vi "Test Repetitive Calls to Next Differnet if Skip.vi"(8 "error in (no error)":errorcluster, 11 "Test Case In":refnum<class "Runnable Next Test.lvclass">) -> (0 "error out":errorcluster, 3 "Test Case Out":refnum<class "Runnable Next Test.lvclass">)   [LabVIEW 2020, in "Runnable Next Test.lvclass"]
uses:
  Runnable Next Test.lvclass
  Runnable Next Test.lvclass/Runnable Next Test.ctl
  Test Doubles/Test Case Test Double/Test Case Test Double.lvclass
  Test Doubles/Test Case Test Double/Methods.ctl
  source/API/LUnit Test Suite/LUnit Test Suite.lvclass
  59278e4f-a81c-4e4b-9980-f8e3984e3fef.vi
  source/API/LUnit Test Case/LUnit Test Case.lvclass
  C:/git/astemes-lunit/source/Core/Runnable/Runnable.lvclass
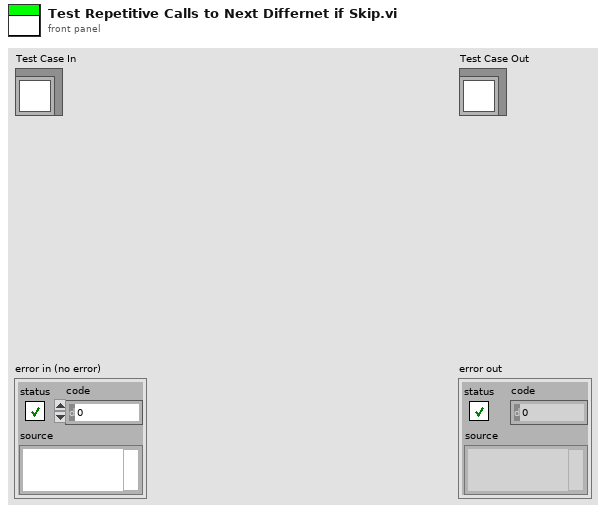
[diagram p1: front panel]
types:
  T1 = typedef "Test Case Test Double.lvclass/Methods.ctl" = enum16{"Test Failing Test.vi", "Test Passing Test.vi", "Test Error Test.vi", "Test Skip Test.vi", "Test Passing Pass If Test.vi", "Test Failing Pass If Test.vi", "Test Failing Fail If Test.vi", "Test Passing Fail If Test.vi", "Test Passing Pass If Error Test.vi", "Test Failing Pass If Error Test.vi", "Test Passing Fail If Error Test.vi", "Test Failing Fail If Error Test.vi", "Test Passing Pass If Equal Test.vi", "Test Failing Pass If Equal Test.vi", "Test Failing Fail If Equal Test.vi", "Test Passing Fail If Equal Test.vi", "Freezing Test.vi"}
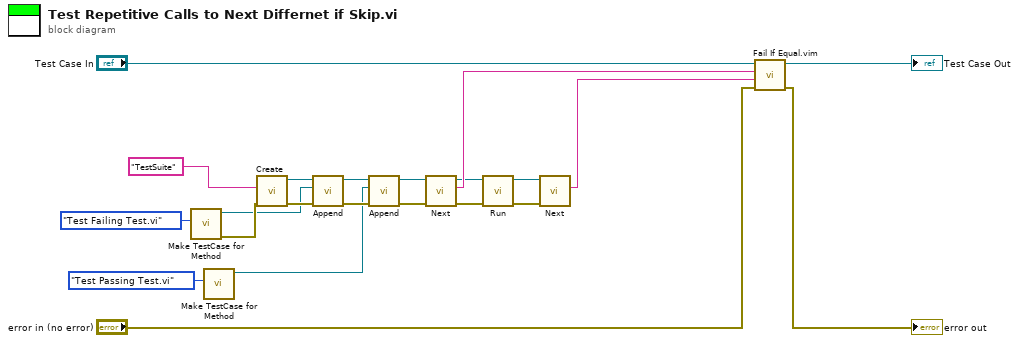
[diagram p0: block diagram]
diagram:
  n1 = call "Make TestCase for Method.vi"("Test Method"=Methods."Test Failing Test.vi") -> ("error out"=w17:errorcluster, "LUnit Test Case V2 out"=w13:refnum<class "LUnit Test Case.lvclass">)  [unwired: 9 in]
  n2 = call "Make TestCase for Method.vi"("Test Method"=Methods."Test Passing Test.vi") -> ("LUnit Test Case V2 out"=w8:refnum<class "LUnit Test Case.lvclass">)  [unwired: 9 in, 1 out]
  n3 = call "Create.vi"("error in (no error)"=w17, "Suite Name"="TestSuite") -> ("error out"=w16:errorcluster, "LUnit Test Suite Out"=w14:refnum<class "LUnit Test Suite.lvclass">)  [unwired: 8 in]
  n4 = call "Append.vi"("error in (no error)"=w16, "Runnable"=w13, "LUnit Test Suite In"=w14) -> ("error out"=w15:errorcluster, "LUnit Test Suite Out"=w9:refnum<class "LUnit Test Suite.lvclass">)  [unwired: 7 in]
  n5 = call "Append.vi"("error in (no error)"=w15, "Runnable"=w8, "LUnit Test Suite In"=w9) -> ("error out"=w10:errorcluster, "LUnit Test Suite Out"=w7:refnum<class "LUnit Test Suite.lvclass">)  [unwired: 7 in]
  n6 = call-dynamic "Next.vi"("error in (no error)"=w10, "LUnit Test Suite In"=w7) -> ("error out"=w4:errorcluster, "Name"=w6:string, "LUnit Test Suite Out"=w2:refnum<class "LUnit Test Suite.lvclass">)  [unwired: 6 in, 1 out]
  n7 = call-dynamic "Run.vi"("error in (no error)"=w4, "LUnit Test Suite In"=w2) -> ("error out"=w3:errorcluster, "LUnit Test Suite In 2"=w1:refnum<class "LUnit Test Suite.lvclass">)  [unwired: 6 in, 2 out]
  n8 = call-dynamic "Next.vi"("error in (no error)"=w3, "LUnit Test Suite In"=w1) -> ("Name"=w5:string)  [unwired: 6 in, 3 out]
  n9 = call "Fail If Equal.vim"("error in (no error)"="error in (no error)", "Actual"=w5, "Expected"=w6, "LUnit Test Case In"="Test Case In") -> ("error out"=→"error out":errorcluster, "LUnit Test Case Out"=→"Test Case Out":refnum<class "Runnable Next Test.lvclass">)  [unwired: 6 in]
